vi "Support_ReadIniFile.vi"(1 "Parameter name":string, 5 "error in (no error)":errorcluster, 6 "Parameter names":string[](array[string]), 8 "Sub test case":string) -> (10 "Timer start":u32, 12 "Parameters as string":string[](array[string]), 14 "Parameter1 as string":string, 15 "Parameter2 as string":string, 16 "Parameter1 as I32":i32, 17 "Parameter2 as I32":i32, 18 "Parameters as I32":i32[](array[numeric]), 19 "error out":errorcluster)   [LabVIEW 2009]
doc: "Reads configuration parameters from file."
uses:
  <vilib>/Utility/config.llb/Read Key (String).vi
  <vilib>/Utility/config.llb/NI_LVConfig.lvlib
  <vilib>/addons/_AddQ/G#Object/G#Object.lvclass
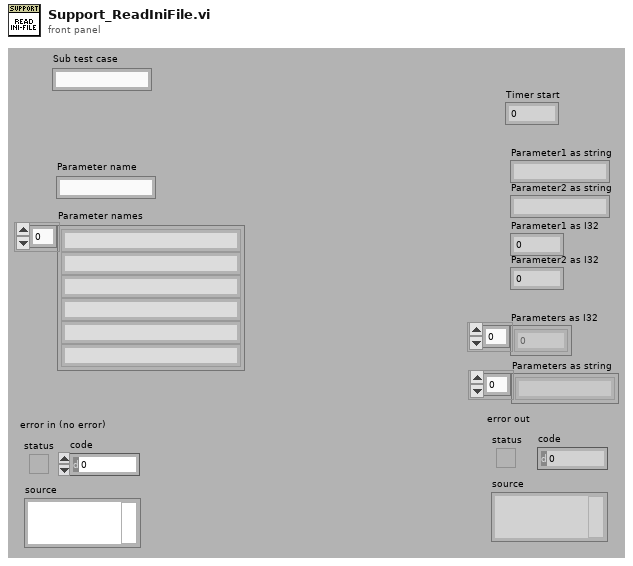
[diagram p1: front panel]
types:
  T1 = typedef "NI_LVConfig.lvlib/Config Data RefNum.ctl" = refnum<k1>
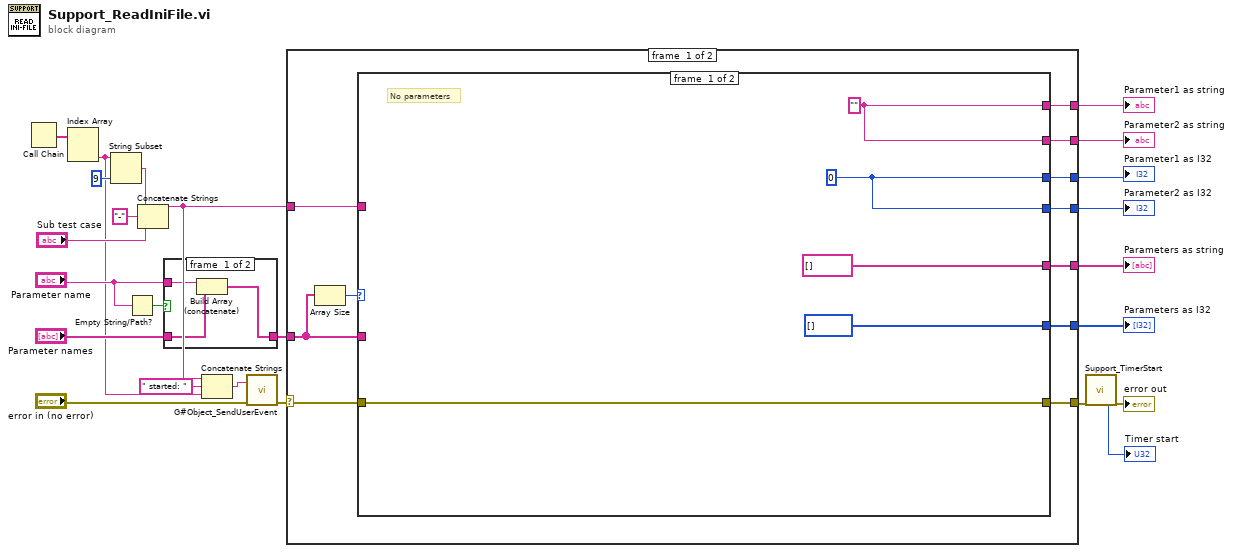
[diagram p0: block diagram]
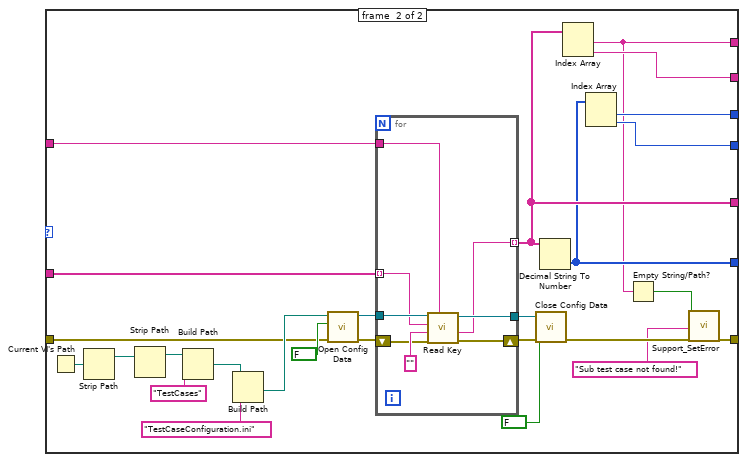
[diagram p3: hidden frame]
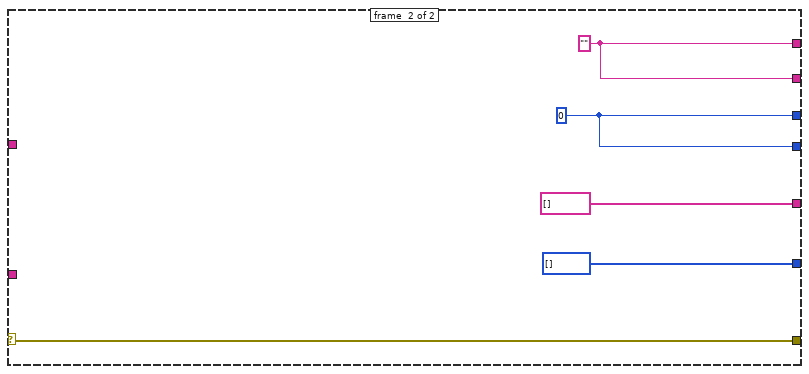
[diagram p4: hidden frame]
diagram:
  n1 = Call Chain() -> (call chain=w9:string[])
  n2 = Index Array(array=w9) -> (element #2=w1:string)  [unwired: 2 in, 1 out]
  n3 = String Subset(string=w1, length (rest)=9 ("length (rest)")) -> (substring=w8:string)  [unwired: 1 in]
  n4 = Empty String/Path?(string/path="Parameter name") -> (empty?=w16:bool)
  n5 = Concatenate Strings(w8, "-", "Sub test case") -> (w3:string)
  n6 = case shown="False" w16 {
    tunnel: [w26 w28] -> w17
    tunnel: "Parameter names" -> [w25 w28]
    tunnel: "Parameter name" -> [w27 _]
    frame #0 {
      n7 = Build Array (concatenate)(w27, w25) -> (w26:string[])
    }
    frame #1 {
    }
  }
  n8 = Concatenate Strings(w3, " started: " ("string"), w1) -> (w4:string)
  n9 = call <vilib>:"G#Object_SendUserEvent.vi"("text"=w4, "error in (no error)"="error in (no error)") -> ("error out"=w5:errorcluster)  [unwired: 16 in, 1 out]
  n10 = case shown="No Error" w5 {
    selector: w5 -> [w37 w81]
    tunnel: w3 -> [w39 _]
    tunnel: [w38 w81] -> w12
    tunnel: [w36 string[] []] -> w24
    tunnel: [w35 i32[] []] -> w23
    tunnel: [w34 w80] -> w22
    tunnel: [w33 w80] -> w21
    tunnel: [w32 w79] -> w20
    tunnel: [w31 w79] -> w19
    tunnel: w17 -> [w30 _]
    frame #0 {
      n11 = Array Size(array=w30) -> (size(s)=w29:i32)
      n12 = case shown="1.., Default" w29 {
        tunnel: w39 -> [_ w68]
        tunnel: [w40 w54] -> w38
        tunnel: w37 -> [w40 w62]
        tunnel: [string[] [] w61] -> w36
        tunnel: [i32[] [] w60] -> w35
        tunnel: [w44 w49] -> w34
        tunnel: [w44 w50] -> w33
        tunnel: [w43 w59] -> w32
        tunnel: [w43 w58] -> w31
        tunnel: w30 -> [_ w57]
        frame #0 {
          w43 = 0 ("value")
          w44 = "" ("value")
          # "No parameters"
        }
        frame #1 {
          n13 = Current VI's Path() -> (path=w47:path)
          n14 = Strip Path(path=w47) -> (stripped path=w45:path)  [unwired: 1 out]
          n15 = Strip Path(path=w45) -> (stripped path=w46:path)  [unwired: 1 out]
          n16 = Build Path(base path=w46, name or relative path="TestCases") -> (appended path=w56:path)
          n17 = Build Path(base path=w56, name or relative path="TestCaseConfiguration.ini") -> (appended path=w64:path)
          n18 = call <vilib>:"Open Config Data.vi"("error in (no error)"=w62, "create file if necessary (T)"=FALSE ("create file if necessary? (T)"), "configuration file path"=w64) -> ("error out"=w70:errorcluster, "refnum"=w69:T1)  [unwired: 6 in, 1 out]
          n19 = for {
            shift-right: [w73] -> w67
            shift-left: w70 -> [w77]
            tunnel: w69 -> [w76]
            tunnel: w57 -> [w75] mode=indexing
            tunnel: w68 -> [w74]
            tunnel: [w72] -> w63
            tunnel: [w71] -> w61 mode=indexing
            n20 = call-poly <vilib>:"Read Key.vi"("section"=w74, "error in (no error)"=w77, "default value"="", "key"=w75, "refnum"=w76) -> ("error out"=w73:errorcluster, "value"=w71:string, "refnum out"=w72:T1)  [unwired: 3 in, 1 out]
          }
          n21 = call <vilib>:"Close Config Data.vi"("error in (no error)"=w67, "write file if changed (T)"=FALSE ("write configuration file? (T)"), "refnum"=w63) -> ("error out"=w53:errorcluster)  [unwired: 7 in, 1 out]
          n22 = Decimal String To Number(string=w61) -> (number=w60:i32[])  [unwired: 2 in, 1 out]
          n23 = Index Array(array=w61) -> (element #1=w49:string, element #2=w50:string)  [unwired: 2 in]
          n24 = Index Array(array=w60) -> (element #1=w59:i32, element #2=w58:i32)  [unwired: 2 in]
          n25 = Empty String/Path?(string/path=w49) -> (empty?=w52:bool)
          n26 = call "Support_SetError.vi"("status"=w52, "source"="Sub test case not found!", "error in (no error)"=w53) -> ("error out"=w54:errorcluster)  [unwired: 16 in]
        }
      }
    }
    frame #1 {
      w79 = 0 ("value")
      w80 = "" ("value")
    }
  }
  "Parameters as I32" <- w23
  "Parameters as string" <- w24
  "Parameter1 as string" <- w22
  "Parameter2 as string" <- w21
  "Parameter1 as I32" <- w20
  "Parameter2 as I32" <- w19
  n27 = call "Support_TimerStart.vi"("error in (no error)"=w12) -> ("Start time"=→"Timer start":u32, "error out"=→"error out":errorcluster)  [unwired: 17 in]
